vi "TEST - Encode Section and Key Names.vi"(8 "error in (no error)":errorcluster) -> (0 "error out":errorcluster, 2 "pass":bool)   [LabVIEW 2020]
uses:
  <userlib>/_OpenG.lib/error/error.llb/openg_error.lvlib
panel:
  out "Failures":T1(array[cluster])
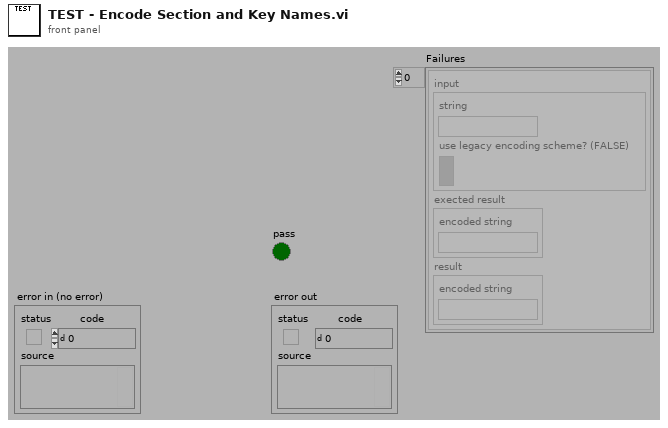
[diagram p1: front panel]
types:
  T1 = cluster{"input":cluster{"string":string, "use legacy encoding scheme? (FALSE)":bool}, "exected result":cluster{"encoded string":string}, "result":cluster{"encoded string":string}}[]
  T2 = cluster{"input":cluster{"string":string, "use legacy encoding scheme? (FALSE)":bool}, "exected result":cluster{"encoded string":string}, "result":cluster{"encoded string":string}}
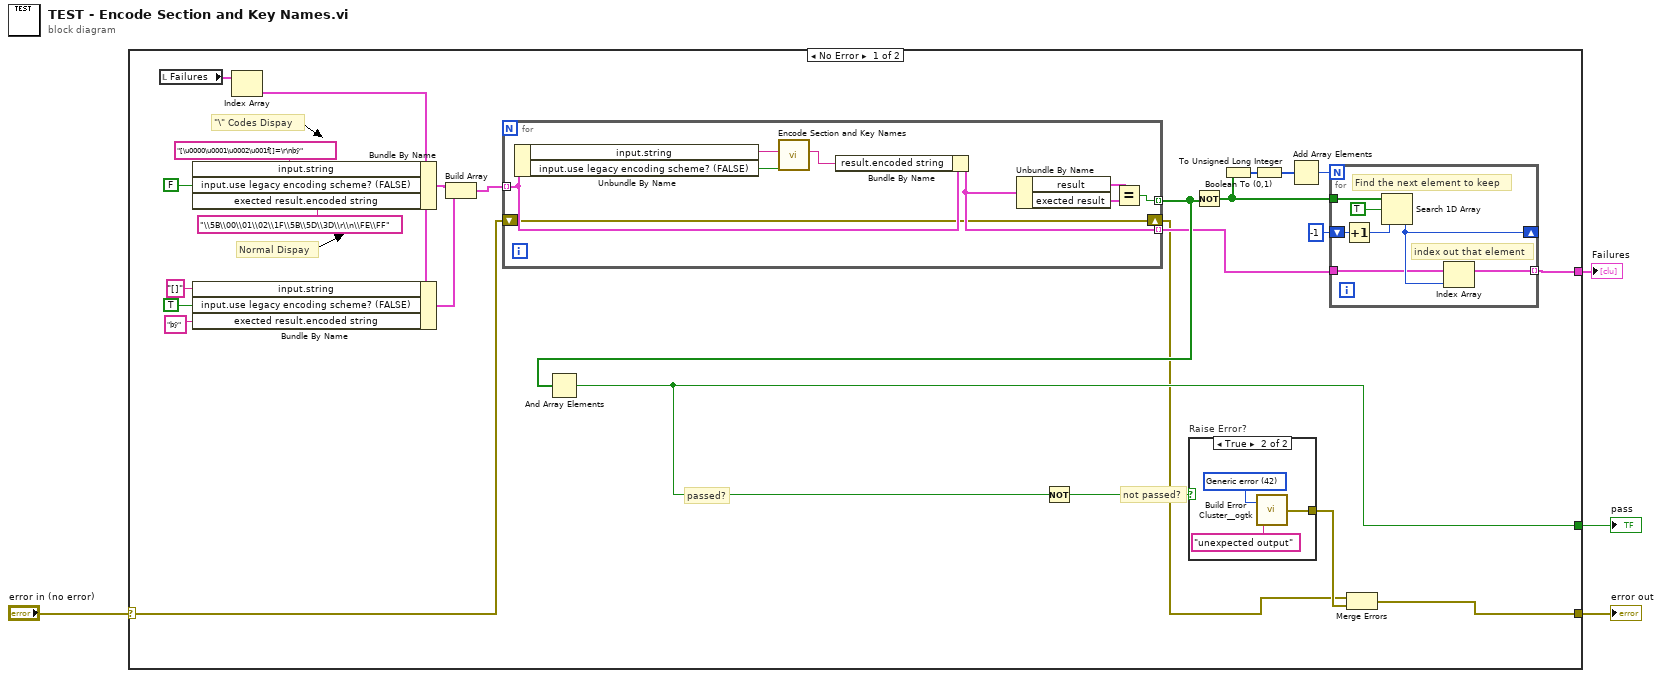
[diagram p0: block diagram]
diagram:
  n1 = case shown="No Error" "error in (no error)" {
    selector: "error in (no error)" -> [w15 w49]
    tunnel: [w26 _] -> w4
    tunnel: [w29 w49] -> w2
    tunnel: [w18 _] -> w1
    frame No Error {
      # "Normal Dispay"
      # "\"\\\" Codes Dispay"
      # "not passed?"
      # "passed?"
      n2 = local read "Failures"() -> (w13:T1)
      n3 = Index Array(array=w13) -> (element=w12:T2)  [unwired: 1 in]
      n4 = Bundle By Name(cluster=w12, "input.string"="[\u0000\u0001\u0002\u001f[]=\r\nþÿ", "input.use legacy encoding scheme? (FALSE)"=FALSE, "exected result.encoded string"="\\5B\\00\\01\\02\\1F\\5B\\5D\\3D\\r\\n\\FE\\FF") -> (w17:T2)
      n5 = Bundle By Name(cluster=w12, "input.string"="[]", "input.use legacy encoding scheme? (FALSE)"=TRUE, "exected result.encoded string"="þÿ") -> (w5:T2)
      n6 = Build Array(w17, w5) -> (w16:T1)
      n7 = for {
        tunnel: w16 -> [w44] mode=indexing
        tunnel: [w45] -> w20 mode=indexing
        tunnel: [w43] -> w19 mode=indexing
        shift-right: [w38] -> w14
        shift-left: w15 -> [w38]
        n8 = Unbundle By Name(w44) -> ("input.string"=w40:string, "input.use legacy encoding scheme? (FALSE)"=w39:bool)
        n9 = call "Encode Section and Key Names.vi"("use legacy encoding scheme? (FALSE)"=w39, "string"=w40) -> ("encoded string"=w37:string)  [unwired: 9 in]
        n10 = Bundle By Name(cluster=w44, "result.encoded string"=w37) -> (w43:T2)
        n11 = Unbundle By Name(w43) -> ("result"=w42:cluster{"encoded string":string}, "exected result"=w41:cluster{"encoded string":string})
        n12 = Equal?(x=w42, y=w41) -> (x = y?=w45:bool)
      }
      n13 = And Array Elements(Boolean array=w20) -> (logical AND=w26:bool)
      n14 = Not(x=w26) -> (.not. x?=w27:bool)
      n15 = case "Raise Error?" shown="True" w27 {
        tunnel: [_ w46] -> w28
        frame False {
        }
        frame True {
          w47 = 42 items=["No error", "Argument error", "Memory is full", "Out of zone", "End of file", "File already open", "Generic file I/O error", "File not found", "File permission error", "Disk is full", "Duplicate path", "Too many files open", "System feature not enabled", "Resource file not found", "Cannot add resource", "Resource not found", "Image not found", "Image memory error", "Pen does not exist", "Config type invalid", "Config token not found", "Config parse error", "Config memory error", "Bad external code format", "Bad external code offset", "External code not present", "Null window", "Destroy window error", "Null menu", "Print aborted", "Bad print record", "Print driver error", "Windows error during printing", "Memory error during printing", "Print dialog error", "Generic print error", "Invalid device refnum", "Device not found", "Device parameter error", "Device unit error", "Cannot open device", "Device call aborted", "Generic error", "Cancelled by user", "Object ID too low", "Object ID too high", "Object not in heap", "Unknown heap", "Unknown object (invalid DefProc)", "Unknown object (DefProc not in table)", "Message out of range", "Invalid (null) method", "Unknown message", "Manager call not supported", "Bad address", "Network operation in progress", "Network operation timed out", "Connection is busy", "Network attribute not supported", "Network error", "Address in use", "System out of memory", "Connection aborted", "Connection refused", "Not connected", "Already connected", "Connection closed", "Initialization error (interapplication manager)", "Bad occurrence", "Wait on unbound occurrence handler", "Occurrence queue overflow", "Datalog type conflict", "Unused", "Unrecognized type (interapplication manager)", "Memory corrupt", "Failed to make temporary DLL", "Old CIN version", "Drag socket not found", "Failed to load drop-object", "Failed to register OLE object", "Failed to release OLE object", "Format specifier type mismatch", "Unknown format specifier", "Too few format specifiers", "Too many format specifiers", "Scan failed", "Newer CIN version", "Error converting to variant", "Runtime menu error", "Password tampered", "Variant attribute not found", "Incompatible variant data type", "Event data is not available", "Event Store is not present", "Occurrence is not found", "Event Queue is not created", "Event info is not available", "Refnum passed is NULL", "Error retrieving Class GUID", "Error retrieving CoClass GUID", "Error retrieving TypeLib GUID.", "Bad built application magic bytes.", "Specific driver is different from the specific driver associated with the Logical Name.", "There is no session opened to the class driver.", "Max Error", "MAX - Error with config objects", "MAX - Error loading configuration", "MAX - Group not supported"]
          n16 = call <userlib>:"Build Error Cluster__ogtk.vi"("String to Prepend to source (\"\")"="unexpected output" ("String to Prepend to source (\"\")"), "code"=w47) -> ("error out"=w46:errorcluster)
        }
      }
      n17 = Not(x=w20) -> (.not. x?=w22:bool[])
      n18 = Boolean To (0,1)(Boolean=w22) -> (0, 1=w23:i16[])
      n19 = To Unsigned Long Integer(number=w23) -> (unsigned 32bit integer=w21:u32[])
      n20 = Add Array Elements(numeric array=w21) -> (sum=w24:u32)
      n21 = for {
        N: w24 -> [_]
        tunnel: w19 -> [w32]
        tunnel: w22 -> [w36]
        shift-right: [w33] -> _
        shift-left: -1 ("start index (0)") -> [w34]
        tunnel: [w31] -> w18 mode=indexing
        # "index out that element"
        # "Find the next element to keep"
        n22 = Increment(x=w34) -> (x+1=w30:i32)
        n23 = Search 1D Array(1D array=w36, element=TRUE, start index (0)=w30) -> (index of element=w33:i32)
        n24 = Index Array(array=w32, index=w33) -> (element=w31:T2)
      }
      n25 = Merge Errors(w14, w28) -> (w29:errorcluster)
    }
    frame Error {
    }
  }
  "pass" <- w4
  "error out" <- w2
  "Failures" <- w1
